vi "test #56.vi"() -> ()   [LabVIEW 2017]
uses:
  INI-Static-Variable-Support/INI-Static-Variable-Support.lvlib
  <userlib>/_NEVSTOP/Communicable State Machine(CSM)/Communicable State Machine.lvlib
panel:
  out "String out":string
  out "Key Found?":bool
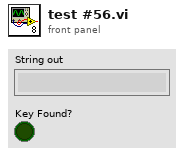
[diagram p1: front panel]
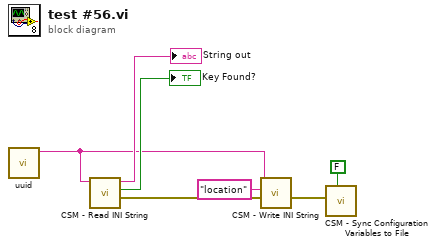
[diagram p0: block diagram]
diagram:
  n1 = call <userlib>:"uuid.vi"() -> ("UUID"=w2:string)  [unwired: 11 in]
  n2 = call "CSM - Read INI String.vi"("String in"=w2) -> ("error out"=w5:errorcluster, "Key Found?"=→"Key Found?":bool, "String out"=→"String out":string)  [unwired: 6 in]
  n3 = call "CSM - Write INI String.vi"("error in (no error)"=w5, "String"="location", ">> Variable Name >>"=w2) -> ("error out"=w4:errorcluster)  [unwired: 5 in, 1 out]
  n4 = call "CSM - Sync Configuration Variables to File.vi"("All Temp Variable to Default Ini(F)"=FALSE, "error in (no error)"=w4) -> ()  [unwired: 7 in, 1 out]
